vi "AlmostEqual.vi"(0 "VI Reference In":refnum<vi>, 1 "Label":string, 2 "delimiter (>>)":string=">>", 3 "Assert Only? (F)":bool, 5 "Control Name":string, 7 "Control Value":ext, 9 "Tolerance":ext=0.00000100000000000000000004, 11 "Error In":errorcluster, 12 "Assert Interval(10 ms)":u32=10, 13 "Timeout(5 sec)":dbl=5.0, 14 "Use Percentage of X (F)":bool) -> (4 "VI Reference Out":refnum<vi>, 15 "Error Out":errorcluster)   [LabVIEW 2016, in "AssertControlValue.lvlib"]
doc: "Asserts if the numeric values of controls are almost equal.\n\nThe input control name is given as a string , incase of path, use delimiters inbetween the path.\nThis VI gets the value of the control, untill the value is almost equal to the input value."
uses:
  AssertControlValue.lvlib
  Setup/GetControlRef/GetControlRefByPath.vi
  <vilib>/addons/_JKI Toolkits/Caraya/classes/Assert/Assert Almost Equal_Float.vi
  <vilib>/addons/_JKI Toolkits/Caraya/classes/Assert/Assert Equal Value_Variant.vi
  <vilib>/addons/_JKI Toolkits/Caraya/classes/Assert/Assert.lvclass
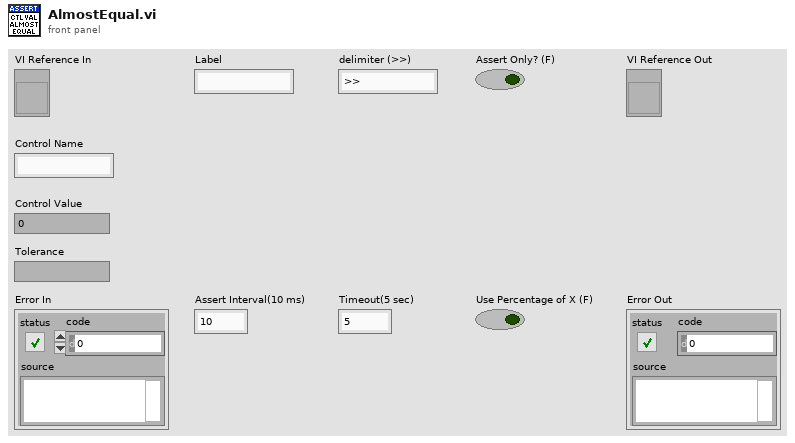
[diagram p1: front panel]
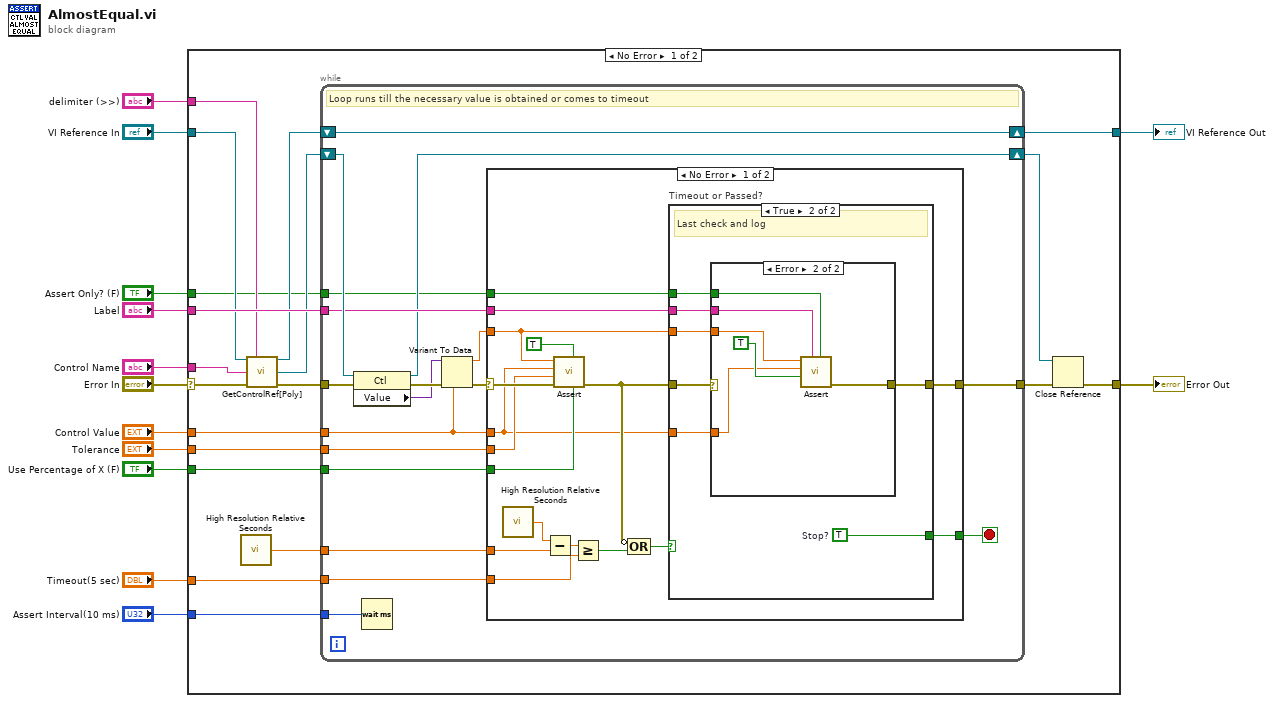
[diagram p0: block diagram]
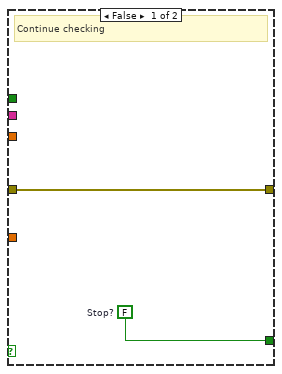
[diagram p2: hidden frame]
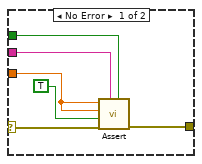
[diagram p3: hidden frame]
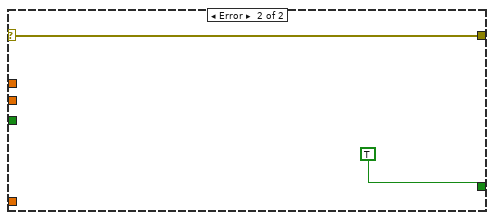
[diagram p4: hidden frame]
diagram:
  n1 = case shown="No Error" "Error In" {
    selector: "Error In" -> [w25 w92]
    tunnel: "Timeout(5 sec)" -> [w32 _]
    tunnel: [w31 w91] -> w12
    tunnel: "Control Value" -> [w30 _]
    tunnel: "Tolerance" -> [w29 _]
    tunnel: [w18 w92] -> w9
    tunnel: "Assert Interval(10 ms)" -> [w27 _]
    tunnel: "Label" -> [w26 _]
    tunnel: "VI Reference In" -> [w24 w91]
    tunnel: "Control Name" -> [w23 _]
    tunnel: "delimiter (>>)" -> [w16 _]
    tunnel: "Use Percentage of X (F)" -> [w15 _]
    tunnel: "Assert Only? (F)" -> [w14 _]
    frame No Error {
      n2 = call <vilib>:"High Resolution Relative Seconds.vi"() -> ("relative seconds"=w22:dbl)
      n3 = call-poly "GetControlRef[Poly].vi"("VI Reference In"=w24, "delimiter (>>)"=w16, "Control Name"=w23, "error In"=w25) -> ("VI Reference Out"=w20:refnum<vi>, "Ctl Refnum"=w19:refnum<vi>, "error out"=w21:errorcluster)  [unwired: 9 in]
      n4 = while {
        tunnel: w30 -> [w44]
        tunnel: w32 -> [w49]
        tunnel: w22 -> [w50]
        tunnel: w21 -> [w42]
        tunnel: [w47] -> w28
        tunnel: w29 -> [w45]
        tunnel: w27 -> [w33]
        tunnel: w26 -> [w37]
        shift-right: [w40] -> w31
        shift-left: w20 -> [w40]
        shift-right: [w36] -> w17
        shift-left: w19 -> [w41]
        tunnel: w15 -> [w35]
        tunnel: w14 -> [w34]
        stop <- w48 stop-if-true
        # "Loop runs till the necessary value is obtained or comes to timeout"
        n5 = property class="Ctl"(reference=w41, error in=w42) -> (reference out=w36:refnum<vi>, error out=w46:errorcluster, "Value"=w39:variant)
        n6 = Wait (ms)(milliseconds to wait=w33) -> ()  [unwired: 1 out]
        n7 = Variant To Data(error in=w46, type=w44, Variant=w39) -> (data=w43:ext, error out=w38:errorcluster)
        n8 = case shown="No Error" w38 {
          selector: w38 -> [w63 w90]
          tunnel: w50 -> [w67 _]
          tunnel: w49 -> [w64 _]
          tunnel: [w57 TRUE] -> w48
          tunnel: [w58 w90] -> w47
          tunnel: w45 -> [w62 _]
          tunnel: w44 -> [w51 _]
          tunnel: w43 -> [w59 _]
          tunnel: w37 -> [w61 _]
          tunnel: w35 -> [w56 _]
          tunnel: w34 -> [w52 _]
          frame No Error {
            n9 = call <vilib>:"High Resolution Relative Seconds.vi"() -> ("relative seconds"=w66:dbl)
            n10 = Subtract(x=w66, y=w67) -> (x-y=w65:dbl)
            n11 = call-poly <vilib>:"Assert.vi"("Use Percentage of X (F)"=w56, "Assert Only? (F)"=TRUE, "error in (no error)"=w63, "Tolerance"=w62, "Y"=w51, "X"=w59) -> ("error out"=w55:errorcluster)  [unwired: 5 in]
            n12 = Greater Or Equal?(x=w65, y=w64) -> (x >= y?=w54:bool)
            n13 = Compound Arithmetic op=OR(invert w55, w54) -> (w53:bool)
            n14 = case "Timeout or Passed?" shown="True" w53 {
              tunnel: w55 -> [w69 w72]
              tunnel: w59 -> [_ w75]
              tunnel: w61 -> [_ w76]
              tunnel: [w69 w71] -> w58
              tunnel: [w68 w74] -> w57
              tunnel: w52 -> [_ w73]
              tunnel: w51 -> [_ w70]
              frame False {
                w68 = FALSE  # Stop?
                # "Continue checking"
              }
              frame True {
                w74 = TRUE  # Stop?
                # "Last check and log"
                n15 = case shown="Error" w72 {
                  selector: w72 -> [w78 _]
                  tunnel: w76 -> [w82 w88]
                  tunnel: w75 -> [w80 w84]
                  tunnel: w73 -> [w81 w87]
                  tunnel: [w77 w86] -> w71
                  tunnel: w70 -> [_ w83]
                  frame No Error {
                    n16 = call-poly <vilib>:"Assert.vi"("Assert Only? (F)"=w81, "Label"=w82, "error in (no error)"=w78, "Register with caller test (F)"=TRUE, "Y"=w80, "X"=w80) -> ("error out"=w77:errorcluster)  [unwired: 5 in]
                  }
                  frame Error {
                    n17 = call-poly <vilib>:"Assert.vi"("Assert Only? (F)"=w87, "Label"=w88, "Register with caller test (F)"=TRUE, "Y"=w83, "X"=w84) -> ("error out"=w86:errorcluster)  [unwired: 6 in]
                  }
                }
              }
            }
          }
          frame Error {
          }
        }
      }
      n18 = Close Reference(reference=w17, error in (no error)=w28) -> (error out=w18:errorcluster)
    }
    frame Error {
    }
  }
  "Error Out" <- w9
  "VI Reference Out" <- w12
